vi "coerce_in_range.vi"(3 "min":i8, 4 "x":i8, 5 "max":i8) -> (1 "coerced x":i8)   [LabVIEW 2009]
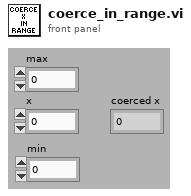
[diagram p1: front panel]
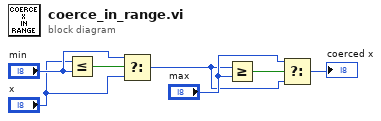
[diagram p0: block diagram]
diagram:
  n1 = Less Or Equal?(x="x", y="min") -> (x <= y?=w7:bool)
  n2 = Select(t="min", s=w7, f="x") -> (s? t:f=w2:i8)
  n3 = Greater Or Equal?(x=w2, y="max") -> (x >= y?=w5:bool)
  n4 = Select(t="max", s=w5, f=w2) -> (s? t:f=→"coerced x":i8)
